vi "ConfigureMeasurementParameters.vi"(0 "NI-DMM in":refnum<class "NI-DMM.lvclass">, 5 "Configure_Parameters":variant, 11 "error in (no error)":errorcluster) -> (4 "NI-DMM out":refnum<class "NI-DMM.lvclass">, 15 "error out":errorcluster)   [LabVIEW 2020, in "AbstractDMM.lvlib" / "NI-DMM.lvclass"]
uses:
  NI-DMM.lvclass
  TypeDef/Configure_Parameters.ctl
  NI-DMM.lvclass/NI-DMM.ctl
  <instrlib>/niDMM/nidmm.llb/niDMM Resolution in Digits.ctl
  <instrlib>/niDMM/nidmm.llb/niDMM Configure Measurement Digits.vi
  Base/AbstractDMM.lvclass
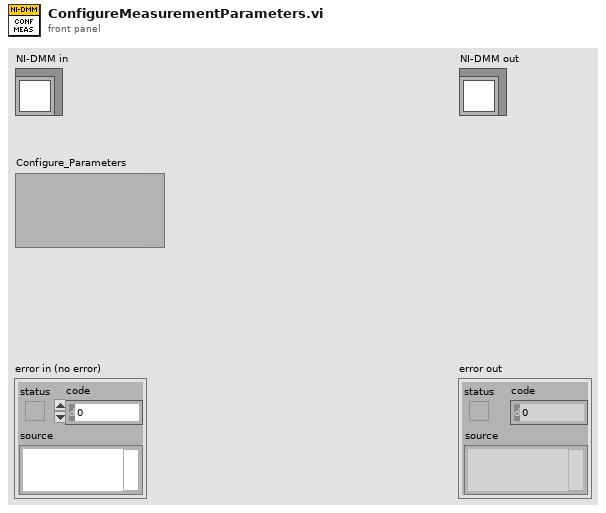
[diagram p1: front panel]
types:
  T1 = typedef "AbstractDMM.lvlib/NI-DMM.lvclass/Configure_Parameters.ctl" = cluster{"Range":dbl, "Measurement Type":enum32{"DC Volts", "AC Volts", "DC Current", "AC Current", "2-wire Resistance", "4-wire Resistance", "Diode", "Frequency", "Period", "AC Volts DC Coupled", "Capacitance", "Inductance", "Temperature"}, "Resolution in Digits":enum32{"3 1/2", "4 1/2", "5 1/2", "6 1/2", "7 1/2"}}
  T2 = enum32{"3 1/2", "4 1/2", "5 1/2", "6 1/2", "7 1/2"}
  T3 = enum32{"DC Volts", "AC Volts", "DC Current", "AC Current", "2-wire Resistance", "4-wire Resistance", "Diode", "Frequency", "Period", "AC Volts DC Coupled", "Capacitance", "Inductance", "Temperature"}
  T4 = typedef "niDMM Resolution in Digits.ctl" = dbl
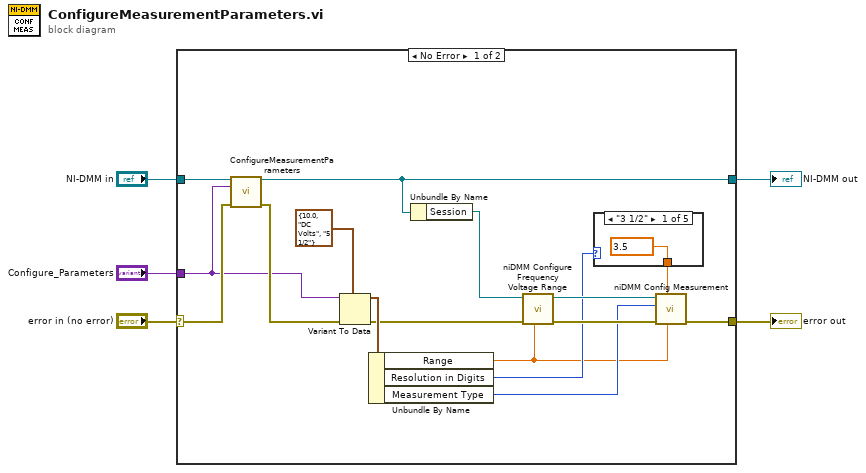
[diagram p0: block diagram]
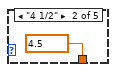
[diagram p2: hidden frame]
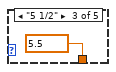
[diagram p3: hidden frame]
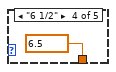
[diagram p4: hidden frame]
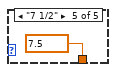
[diagram p5: hidden frame]
diagram:
  n1 = case shown="No Error" "error in (no error)" {
    selector: "error in (no error)" -> [w20 w27]
    tunnel: "NI-DMM in" -> [w21 w28]
    tunnel: "Configure_Parameters" -> [w17 _]
    tunnel: [w13 w27] -> w2
    tunnel: [w12 w28] -> w1
    frame No Error {
      n2 = call-parent "ConfigureMeasurementParameters.vi"("AbstractDMM in"=w21, "Configure_Parameters"=w17, "error in (no error)"=w20) -> ("AbstractDMM out"=w12:refnum<class "NI-DMM.lvclass">, "error out"=w19:errorcluster)  [unwired: 11 in]
      n3 = Variant To Data(error in=w19, type=T1 {"Range"=10.0, "Measurement Type"=enum."DC Volts", "Resolution in Digits"=enum."5 1/2"} ("Configure_Parameters"), Variant=w17) -> (data=w15:T1, error out=w14:errorcluster)
      n4 = Unbundle By Name(w15) -> ("Range"=w6:dbl, "Resolution in Digits"=w7:T2, "Measurement Type"=w8:T3)
      n5 = Unbundle By Name(w12) -> ("Session"=w11:refnum<k15>)
      n6 = call <instrlib>:"niDMM Configure Frequency Voltage Range.vi"("Frequency Voltage Range"=w6, "error in (no error)"=w14, "instrument handle"=w11) -> ("error out"=w18:errorcluster, "instrument handle out"=w10:refnum<k15>)  [unwired: 7 in]
      n7 = case shown="\"3 1/2\"" w7 {
        tunnel: [w22 w23 w24 w25 w26] -> w9
        frame "3 1/2" {
          w22 = T4 3.5 items=["3 1/2"=3.5, "4 1/2"=4.5, "5 1/2"=5.5, "6 1/2"=6.5, "7 1/2"=7.5] ("Resolution in Digits")
        }
        frame "4 1/2" {
          w23 = T4 4.5 items=["3 1/2"=3.5, "4 1/2"=4.5, "5 1/2"=5.5, "6 1/2"=6.5, "7 1/2"=7.5] ("Resolution in Digits")
        }
        frame "5 1/2" {
          w24 = T4 5.5 items=["3 1/2"=3.5, "4 1/2"=4.5, "5 1/2"=5.5, "6 1/2"=6.5, "7 1/2"=7.5] ("Resolution in Digits")
        }
        frame "6 1/2" {
          w25 = T4 6.5 items=["3 1/2"=3.5, "4 1/2"=4.5, "5 1/2"=5.5, "6 1/2"=6.5, "7 1/2"=7.5] ("Resolution in Digits")
        }
        frame "7 1/2" {
          w26 = T4 7.5 items=["3 1/2"=3.5, "4 1/2"=4.5, "5 1/2"=5.5, "6 1/2"=6.5, "7 1/2"=7.5] ("Resolution in Digits")
        }
      }
      n8 = call-poly <instrlib>:"niDMM Config Measurement.vi"("Range"=w6, "Resolution in Digits"=w9, "error in (no error)"=w18, "Function"=w8, "instrument handle"=w10) -> ("error out"=w13:errorcluster)  [unwired: 5 in, 1 out]
    }
    frame Error {
    }
  }
  "error out" <- w2
  "NI-DMM out" <- w1
